vi "myRIO__TCP_constants_byteRange_messageType__getType.vi"(11 "input_byte":u8) -> (3 "output_messageType":u8)   [LabVIEW 2014]
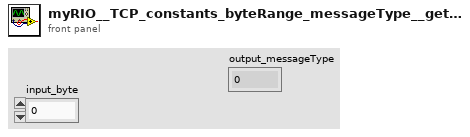
[diagram p1: front panel]
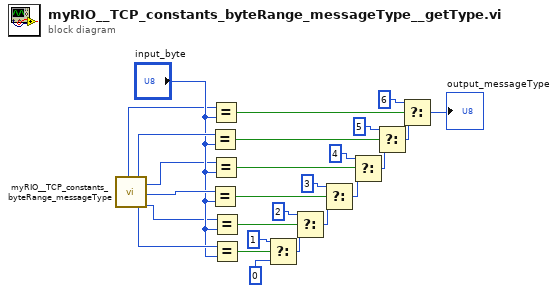
[diagram p0: block diagram]
diagram:
  n1 = call "myRIO__TCP_constants_byteRange_messageType.vi"() -> ("output_Start_byte"=w22:u8, "output_Quit_byte"=w26:u8, "output_analogInput_byte"=w24:u8, "output_Block_byte"=w20:u8, "output_Trial_byte"=w25:u8, "output_selectResponse_byte"=w21:u8)  [unwired: 8 in, 6 out]
  n2 = Equal?(x=w26, y="input_byte") -> (x = y?=w19:bool)
  n3 = Equal?(x=w25, y="input_byte") -> (x = y?=w13:bool)
  n4 = Equal?(x=w22, y="input_byte") -> (x = y?=w18:bool)
  n5 = Equal?(x=w20, y="input_byte") -> (x = y?=w14:bool)
  n6 = Equal?(x=w21, y="input_byte") -> (x = y?=w11:bool)
  n7 = Equal?(x=w24, y="input_byte") -> (x = y?=w9:bool)
  n8 = Select(t=u8 1, s=w9, f=u8 0) -> (s? t:f=w10:u8)
  n9 = Select(t=u8 2, s=w11, f=w10) -> (s? t:f=w12:u8)
  n10 = Select(t=u8 3, s=w13, f=w12) -> (s? t:f=w15:u8)
  n11 = Select(t=u8 4, s=w14, f=w15) -> (s? t:f=w16:u8)
  n12 = Select(t=u8 5, s=w19, f=w16) -> (s? t:f=w17:u8)
  n13 = Select(t=u8 6, s=w18, f=w17) -> (s? t:f=→"output_messageType":u8)
